vi "xyz-dh_localisation.vi"(4 "mid_rng":dbl, 6 "calculate z?":bool, 8 "R":dbl, 9 "weights":dbl[](array[numeric]), 10 "B points":dbl[][](array[numeric])=[[5.0, 3.0], [6.0, 6.0]], 11 "A points":dbl[][](array[numeric])=[[0.0, 1.0], [2.0, 3.0]]) -> (2 "dR":dbl[](array[numeric]), 3 "XYZ":dbl[](array[numeric]))   [LabVIEW 2015]
doc: "INPUT\nR - radius of the window (should be >0.5)\nA points - 2xN array of first points that define lines\nB points - 2xN array of second points that define lines\nw - weights (1D array)\nmid_rng - indication of mid-range angle of rotation in degrees [-180..180]\n\nOUTPUT\nXYZ - x,y position of the particle in pixels (for original image), z-value\ndR - distance from the center to each line (1D vector)\n\nThis vi calculates XYZ position of the in double-helix PSF based microscopy. XY is found as a least square intersection point of gradient lines. For z-value calculation only a A-points (centers of the selected pixels) are used. The gradient image of the double-helix PSF should resemble an ellipse (by adjusting R and threshold). z-value corrseponds to an angle of the ellipse. To bring detected angles in line with calibration a mid_rng parameter is used. It specifies the middle of the rotation range (i.e. the detected angle will be continuous in the range [mid_rng-90, mid_rng+90] )\n\nAuthor: Anatolii Kashchuk"
panel:
  # "This vi finds centroid and z-value from the image of a particle\n\nAuthor: Anatolii Kashchuk"
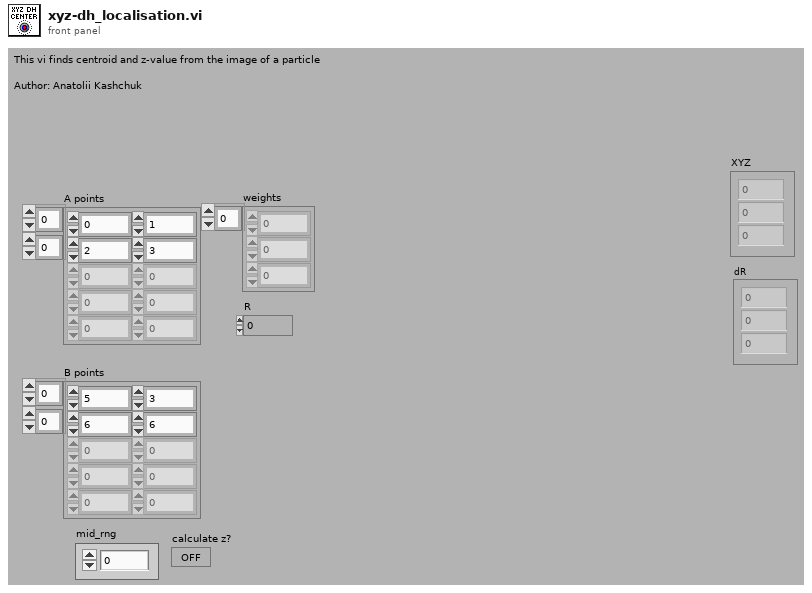
[diagram p1: front panel]
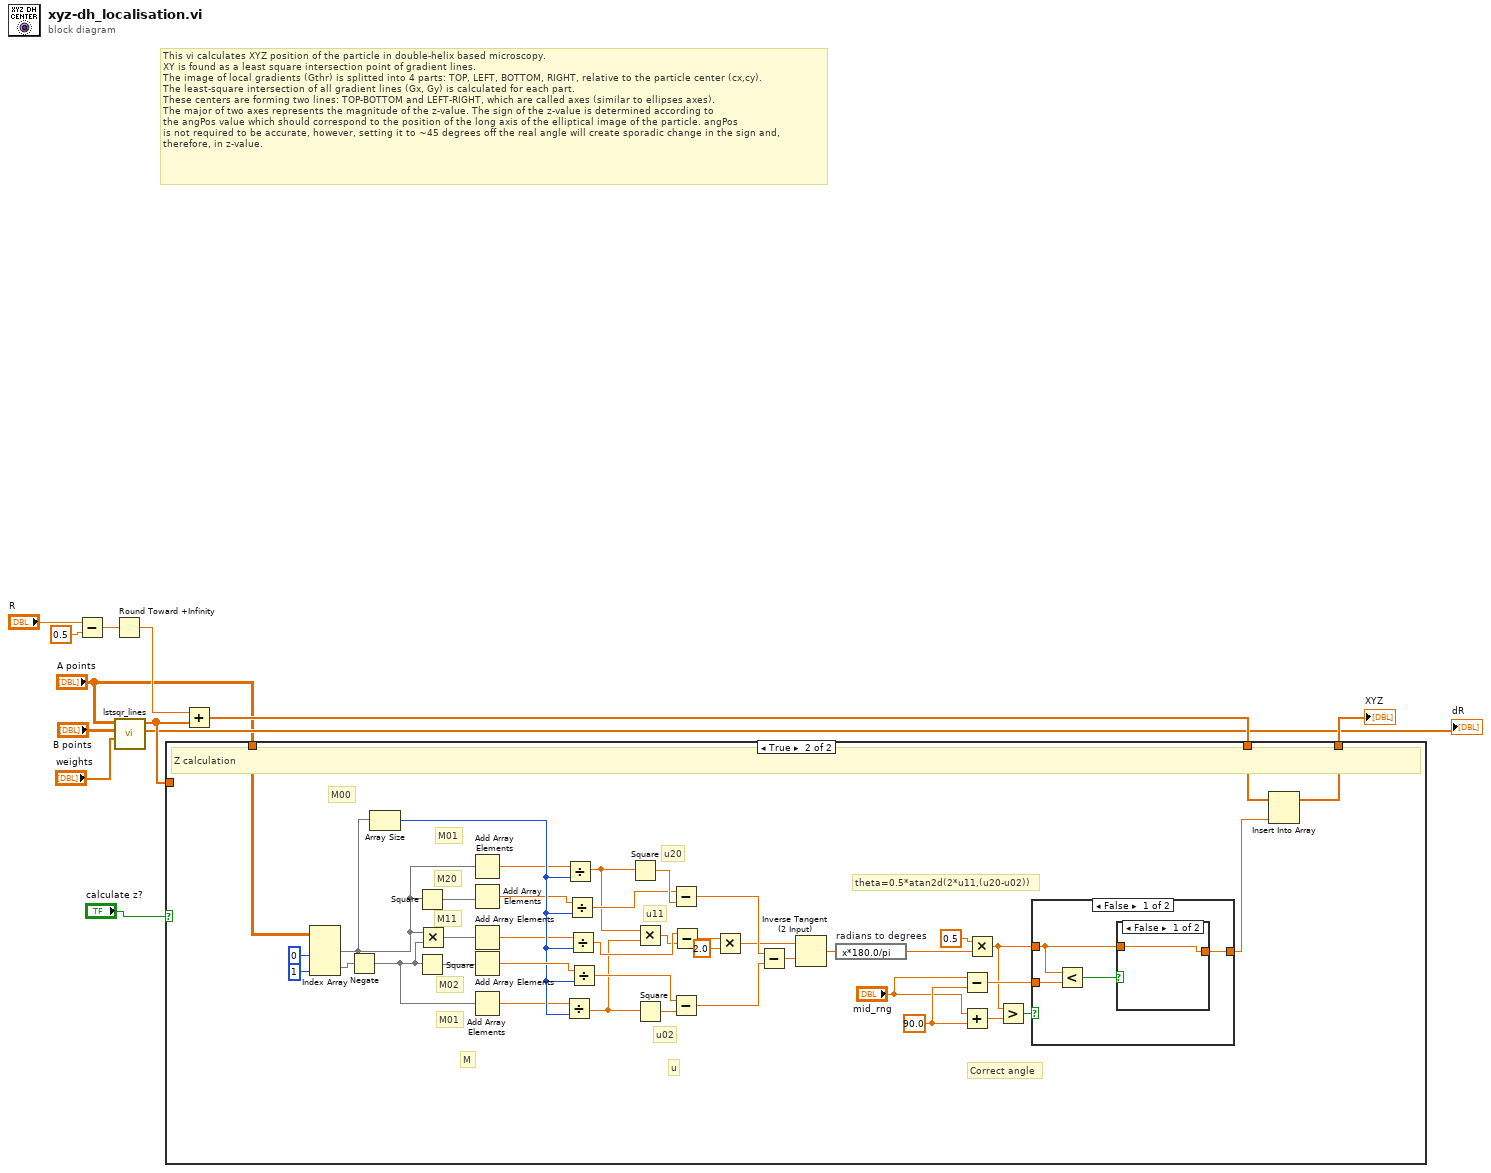
[diagram p0: block diagram]
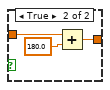
[diagram p3: hidden frame]
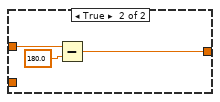
[diagram p4: hidden frame]
diagram:
  # "This vi calculates XYZ position of the particle in double-helix based microscopy. \nXY is found as a least square intersection point of gradient lines. \nThe image of local gradients (Gthr) is splitted into 4 parts: TOP, LEFT, BOTTOM, RIGHT, relative to the particle center (cx,cy). \nThe least-square intersection of all gradient lines (Gx, Gy) is calculated for each part. \nThese centers are forming two lines: TOP-BOTTOM and LEFT-RIGHT, which are called axes (similar to ellipses axes). \nThe major of two axes represents the magnitude of the z-value. The sign of the z-value is determined according to \nthe angPos value which should correspond to the position of the long axis of the elliptical image of the particle. angPos\nis not required to be accurate, however, setting it to ~45 degrees off the real angle will create sporadic change in the sign and, \ntherefore, in z-value."
  n1 = Subtract(x="R", y=0.5) -> (x-y=w8:dbl)
  n2 = Round Toward +Infinity(x=w8) -> (ceil(x): smallest int >= x=w9:dbl)
  n3 = call "lstsqr_lines.vi"("weights"="weights", "B points"="B points", "A points"="A points") -> ("dR"=→"dR":dbl[], "center"=w6:dbl[])  [unwired: 6 in, 1 out]
  n4 = Add(x=w9, y=w6) -> (x+y=w5:dbl[])
  n5 = case shown="True" "calculate z?" {
    tunnel: w6 -> [_ _]
    tunnel: w5 -> [w13 w53]
    tunnel: [w13 w54] -> w4
    tunnel: "A points" -> [_ w17]
    frame False {
    }
    frame True {
      w48 = 90.0 ("y")
      # "u02"
      # "u20"
      # "u11"
      # "M"
      # "theta=0.5*atan2d(2*u11,(u20-u02))"
      # "Correct angle"
      # "M02"
      # "M01"
      # "M20"
      # "M00"
      # "u"
      # "M11"
      # "M01"
      # "Z calculation"
      n6 = Index Array(array=w17, index (col) #1=0 ("disabled index (col)"), index (col) #2=1 ("index (col)")) -> (element #1=w25:dbl[], element #2=w20:dbl[])  [unwired: 2 in]
      n7 = Negate(x=w20) -> (-x=w24:dbl[])
      n8 = Array Size(array=w25) -> (size(s)=w30:i32)
      n9 = Square(x=w25) -> (x^2=w22:dbl[])
      n10 = Square(x=w24) -> (x^2=w21:dbl[])
      n11 = Multiply(x=w25, y=w24) -> (x*y=w23:dbl[])
      n12 = Add Array Elements(numeric array=w25) -> (sum=w27:dbl)
      n13 = Add Array Elements(numeric array=w22) -> (sum=w29:dbl)
      n14 = Add Array Elements(numeric array=w23) -> (sum=w28:dbl)
      n15 = Add Array Elements(numeric array=w21) -> (sum=w31:dbl)
      n16 = Add Array Elements(numeric array=w24) -> (sum=w26:dbl)
      n17 = Divide(x=w26, y=w30) -> (x/y=w33:dbl)
      n18 = Divide(x=w27, y=w30) -> (x/y=w32:dbl)
      n19 = Divide(x=w29, y=w30) -> (x/y=w34:dbl)
      n20 = Divide(x=w28, y=w30) -> (x/y=w39:dbl)
      n21 = Divide(x=w31, y=w30) -> (x/y=w37:dbl)
      n22 = Square(x=w32) -> (x^2=w35:dbl)
      n23 = Multiply(x=w32, y=w33) -> (x*y=w38:dbl)
      n24 = Square(x=w33) -> (x^2=w36:dbl)
      n25 = Subtract(x=w34, y=w35) -> (x-y=w44:dbl)
      n26 = Subtract(x=w37, y=w36) -> (x-y=w45:dbl)
      n27 = Subtract(x=w39, y=w38) -> (x-y=w40:dbl)
      n28 = Multiply(x=w40, y=2.0) -> (x*y=w42:dbl)
      n29 = Subtract(x=w44, y=w45) -> (x-y=w46:dbl)
      n30 = Inverse Tangent (2 Input)(1:w46, 2:w42) -> (0:w15:dbl)
      n31 = expression code="x*180.0/pi" "radians to degrees"(w15) -> (w14:dbl)
      n32 = Subtract(x="mid_rng", y=w48) -> (x-y=w52:dbl)
      n33 = Add(x="mid_rng", y=w48) -> (x+y=w49:dbl)
      n34 = Multiply(x=0.5 ("y"), y=w14) -> (x*y=w51:dbl)
      n35 = Greater?(x=w51, y=w49) -> (0:w50:bool)
      n36 = case shown="False" w50 {
        tunnel: w51 -> [w56 w64]
        tunnel: [w55 w63] -> w16
        tunnel: w52 -> [w57 _]
        frame False {
          n37 = Less?(x=w56, y=w57) -> (x < y?=w58:bool)
          n38 = case shown="False" w58 {
            tunnel: w56 -> [w59 w61]
            tunnel: [w59 w60] -> w55
            frame False {
            }
            frame True {
              n39 = Add(x=w61, y=180.0) -> (x+y=w60:dbl)
            }
          }
        }
        frame True {
          n40 = Subtract(x=w64, y=180.0) -> (x-y=w63:dbl)
        }
      }
      n41 = Insert Into Array(array=w53, new element=w16) -> (w54:dbl[])  [unwired: 1 in]
    }
  }
  "XYZ" <- w4
